vi "Write IMAQdx Session.vi"(8 "error in (no error)":errorcluster, 10 "IMAQdx Session":T1, 11 "Camera Settings Dialog in":refnum<class "Camera Quick Settings Panel.lvclass">) -> (0 "error out":errorcluster, 3 "Camera Settings Dialog out":refnum<class "Camera Quick Settings Panel.lvclass">)   [LabVIEW 2014, in "Camera Quick Settings Panel.lvlib" / "Camera Quick Settings Panel.lvclass"]
uses:
  Camera Quick Settings Panel.lvclass
  <vilib>/userdefined/High Color/IMAQdx.ctl
  Camera Quick Settings Panel.lvclass/Camera Quick Settings Panel.ctl
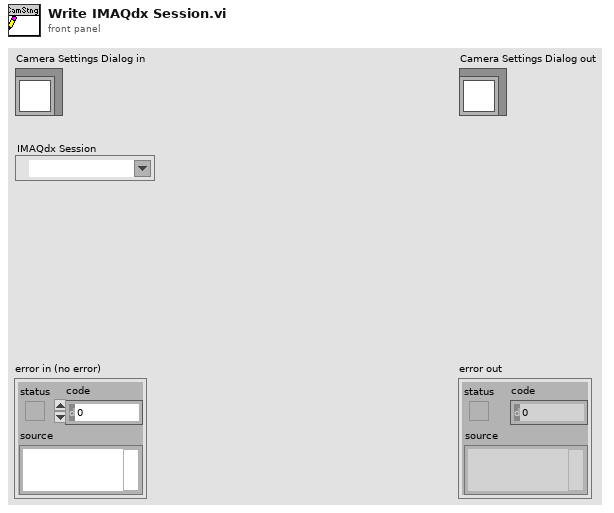
[diagram p1: front panel]
types:
  T1 = typedef "IMAQdx.ctl" = refnum<k21>
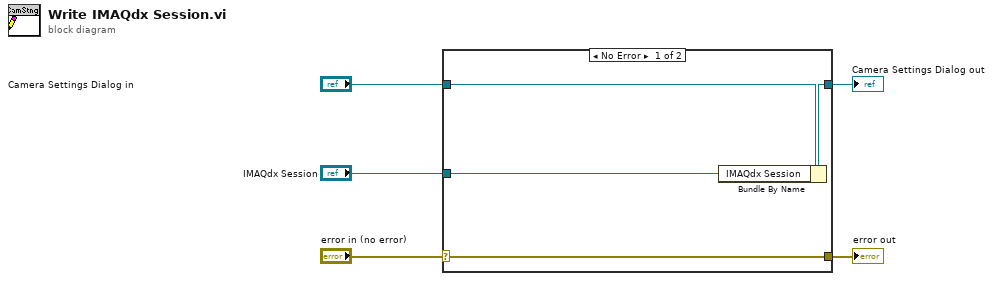
[diagram p0: block diagram]
diagram:
  n1 = case shown="No Error" "error in (no error)" {
    selector: "error in (no error)" -> [w9 w10]
    tunnel: [w9 w10] -> w4
    tunnel: [w7 w11] -> w2
    tunnel: "Camera Settings Dialog in" -> [w8 w11]
    tunnel: "IMAQdx Session" -> [w6 _]
    frame No Error {
      n2 = Bundle By Name(cluster=w8, "IMAQdx Session"=w6) -> (w7:refnum<class "Camera Quick Settings Panel.lvclass">)
    }
    frame Error {
    }
  }
  "error out" <- w4
  "Camera Settings Dialog out" <- w2
